vi "gh-cli Issue List.vi"(8 "error in (no error)":errorcluster, 10 "Options":string, 11 "Git in":refnum<class "Git.lvclass">) -> (0 "error out":errorcluster, 2 "Issues":string, 3 "Git out":refnum<class "Git.lvclass">)   [LabVIEW 2019, in "Git.lvclass"]
doc: "gh issue list [<b>Options</b>]: List issues in a GitHub repository\n\n<b>Options</b>\n--app <string>: Filter by GitHub App author\n-a, --assignee <string>: Filter by assignee\n-A, --author <string>: Filter by author\n-q, --jq <expression>: Filter JSON output using a jq expression\n--json <fields>: Output JSON with the specified fields\n-l, --label <strings>: Filter by label\n-L, --limit <int>: Maximum number of issues to fetch\n--mention <string>: Filter by mention\n-m, --milestone <string>: Filter by milestone number or title\n-S, --search <query>: Search issues with query\n-s, --state <string>: Filter by state: {open|closed|all}\n-t, --template <string>: Format JSON output using a Go template\n-w, --web: List issues in the web browser\n-R, --repo <[HOST/]OWNER/REPO>: Select another repository using the [HOST/]OWNER/REPO format \n\nhttps://cli.github.com/manual/"
uses:
  Git.lvclass
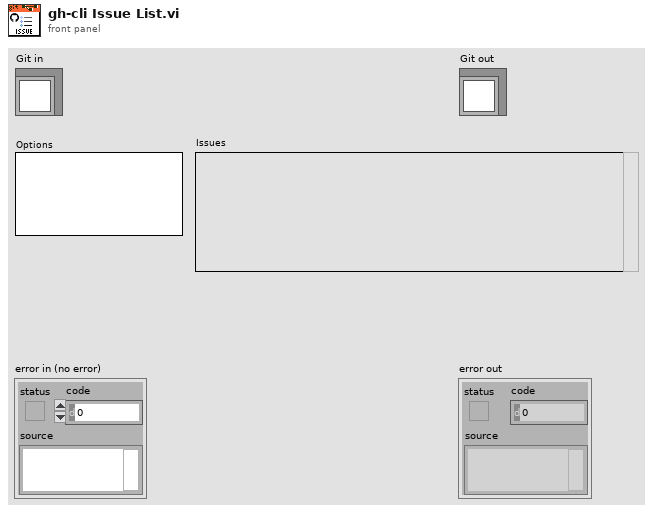
[diagram p1: front panel]
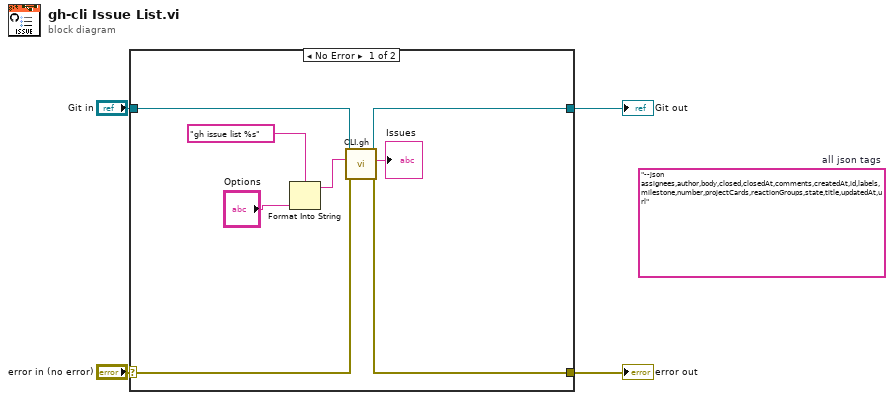
[diagram p0: block diagram]
diagram:
  (unwired) "--json assignees,author,body,closed,closedAt,comments,createdAt,id,labels,milestone,number,projectCards,reactionGroups,state,title,updatedAt,url"  # all json tags
  n1 = case shown="No Error" "error in (no error)" {
    selector: "error in (no error)" -> [w10 w14]
    tunnel: [w9 w14] -> w3
    tunnel: [w11 w13] -> w1
    tunnel: "Git in" -> [w12 w13]
    frame No Error {
      n2 = Format Into String(format string="gh issue list %s" ("Command"), "Options") -> (resulting string=w5:string)  [unwired: 2 in, 1 out]
      n3 = call "CLI.gh.vi"("error in (no error)"=w10, "Command"=w5, "Git in"=w12) -> ("error out"=w9:errorcluster, "standard output"=→"Issues":string, "Git out"=w11:refnum<class "Git.lvclass">)  [unwired: 4 in, 2 out]
    }
    frame Error {
    }
  }
  "error out" <- w3
  "Git out" <- w1
